vi "not found message.vi"(10 "found":bool[](array[boolean]), 11 "paths in":path[](array[path])) -> ()   [LabVIEW 2013]
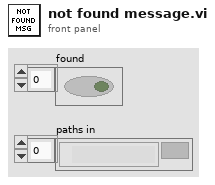
[diagram p1: front panel]
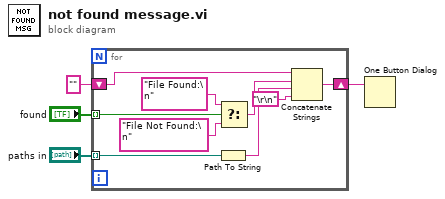
[diagram p0: block diagram]
diagram:
  n1 = for {
    tunnel: "paths in" -> [w9] mode=indexing
    tunnel: "found" -> [w8] mode=indexing
    shift-right: [w7] -> w4
    shift-left: "" -> [w6]
    n2 = Path To String(path=w9) -> (string=w10:string)
    n3 = Select(t="File Found:\n", s=w8, f="File Not Found:\n") -> (s? t:f=w12:string)
    n4 = Concatenate Strings(w6, w12, w10, "\r\n") -> (w7:string)
  }
  n5 = One Button Dialog(message=w4) -> ()  [unwired: 1 in, 1 out]
